vi "ATSh_SetExternalTrigger.vi"(9 "Range":u32, 10 "Coupling":u32, 11 "Handle":u32) -> (0 "Return":u32, 3 "Handle_Out":u32)   [LabVIEW 2015]
doc: "_____AlazarTech, Scope_____\n\nConfigure the External Trigger circuitry.\nHandle input.\n\nCoupling:\n - AC 0x001\n - DC 0x002\n\nRange:\n - DIV5 : 0x000\n - X1 : 0x001"
uses:
  ATSApi.dll
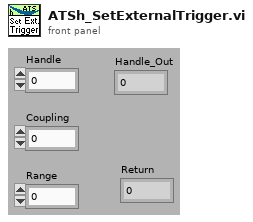
[diagram p1: front panel]
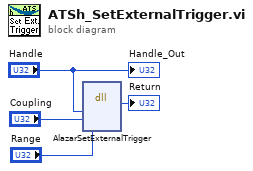
[diagram p0: block diagram]
diagram:
  n1 = dll-call lib="C:/IntensityOCT/trunk/ATSApi.dll" fn="AlazarSetExternalTrigger"("h"="Handle", "Coupling"="Coupling", "Range"="Range") -> (→"Return":u32)  [unwired: 6 in, 2 out]
  "Handle_Out" <- "Handle"
